vi "test_LoadCommandlineArgs_DefaultCase.vi"() -> (3 "Pass?":bool)   [LabVIEW 2019, in "Tests.SolutionBuilder.lvlib"]
uses:
  Tests.SolutionBuilder.lvlib
  SolutionBuilder/Community/Options.ctl
  SolutionBuilder/SolutionBuilder.lvclass
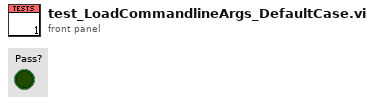
[diagram p1: front panel]
types:
  T1 = typedef "SolutionBuilder.lvlib/SolutionBuilder.lvclass/Options.ctl" = cluster{"Path":path, "Preview?":bool, "Quiet?":bool, "Log file":path, "Success file":path, "Rebuild?":bool, "Keep split projects?":bool}
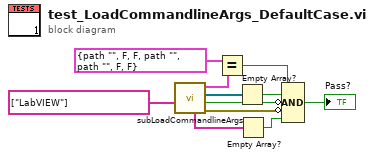
[diagram p0: block diagram]
diagram:
  n1 = call "subLoadCommandlineArgs.vi"("App.Args"=string[] ["LabVIEW"]) -> ("error out"=w11:errorcluster, "From command line?"=w9:bool, "Pre-built libraries"=w6:refnum<class "ProjectItem.lvclass">[], "Options"=w4:T1, "Active targets"=w2:string[])  [unwired: 6 in]
  n2 = Equal?(x=T1 {"Path"=path "", "Preview?"=FALSE, "Quiet?"=FALSE, "Log file"=path "", "Success file"=path "", "Rebuild?"=FALSE, "Keep split projects?"=FALSE} ("Options"), y=w4) -> (x = y?=w8:bool)
  n3 = Empty Array?(array=w6) -> (empty?=w7:bool)
  n4 = Empty Array?(array=w2) -> (empty?=w1:bool)
  n5 = Compound Arithmetic op=AND(w8, w7, invert w9, invert w11, w1) -> (→"Pass?":bool)
